vi "Open.vi"(8 "Error In":errorcluster, 11 "Keithley 6482 In":refnum<visa-resource-name>) -> (0 "Error Out":errorcluster, 3 "Keithley 6482 Out":refnum<visa-resource-name>)   [LabVIEW 8.6, in "Keithley-6482-Visa.lvlib"]
uses:
  Keithley-6482-Visa.lvlib
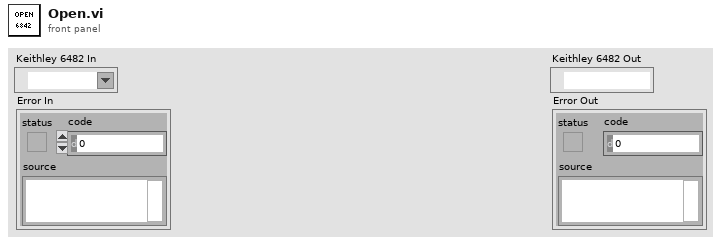
[diagram p1: front panel]
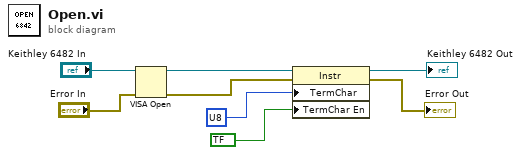
[diagram p0: block diagram]
diagram:
  n1 = VISA Open(error in (no error)="Error In", VISA resource name="Keithley 6482 In") -> (VISA resource name=w6:refnum<visa-resource-name>, error out=w3:errorcluster)  [unwired: 3 in]
  n2 = property class="Instr"(reference=w6, error in=w3, "TermChar"=u8 ? ("Message Based Settings:Termination Character"), "TermChar En"=bool ? ("Message Based Settings:Termination Character Enable")) -> (reference out=→"Keithley 6482 Out":refnum<visa-resource-name>, error out=→"Error Out":errorcluster)
